vi "CSM-MassData Cache Status Viewer.vi"() -> ()   [LabVIEW 2017]
doc: "CSM Massdata cache status viewing tool that allows for an intuitive view of Massdata cache usage, helping to debug and optimize cache configuration.\n\n\n> [!NOTE] <b>CSM Massdata Argument Support</b>\n>\n> CSM Massdata argument support provides an efficient argument passing mechanism for transferring large amounts of data within CSM. By using a memory-efficient reference mechanism instead of direct data transfer, CSM Massdata improves the efficiency and performance of argument passing.\n> - The argument type defined by CSM Massdata is `<MassData>`, which can be obtained using the CSM - Argument Type VI.\n> - Data transmission of CSM Massdata is completely lossless. However, it is not suitable for storing data that requires indefinite persistence.\n>\n> <b>Note</b>: CSM Massdata internally uses a circular buffer mechanism. All CSM modules within the same application share the same Massdata buffer space. When the buffer is full, new data will overwrite old data starting from the beginning. Therefore, you need to set a reasonable buffer size to ensure that data is not overwritten before use, avoiding data loss."
uses:
  addons/MassData-Parameter/_support/FGV-MassData(lvlibp).vi
  addons/MassData-Parameter/CSM MassData Parameter Support.lvlib
panel:
  in  "CacheSize(Byte)":u32 format="%.0p"
  in  "Remove all Configurations":bool
  out "Write":cluster{dbl, dbl}(slide)={287840.0, 276144.0} scale=1.0..100000000.0 scale format="%#_6p"
  out "Read":cluster{dbl, dbl}(slide)={287840.0, 276144.0} scale=1.0..100000000.0 scale format="%#_6p"
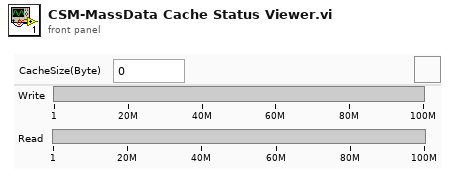
[diagram p1: front panel]
types:
  T1 = typedef "CSM MassData Parameter Support.lvlib/Def-MassDataOper-Status.ctl" = cluster{"Start":i32, "Size":i32, "Total":i32}
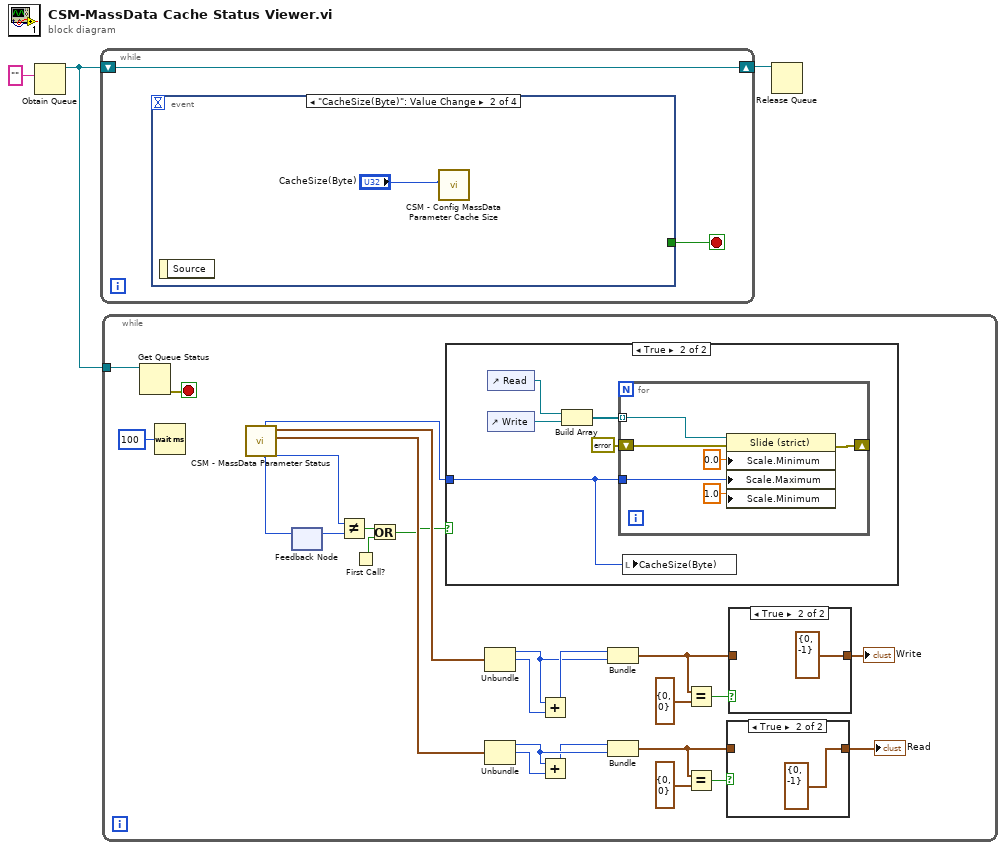
[diagram p0: block diagram]
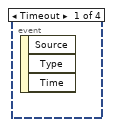
[diagram p2: hidden frame]
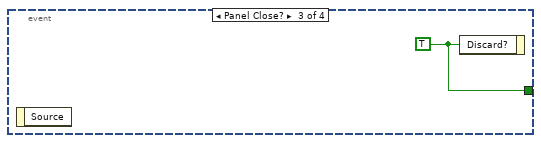
[diagram p3: hidden frame]
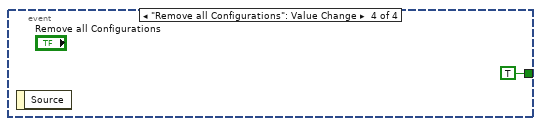
[diagram p4: hidden frame]
diagram:
  n1 = Obtain Queue(element data type="" ("name (unnamed)")) -> (queue out=w3:refnum<queue>)  [unwired: 4 in, 2 out]
  n2 = while {
    shift-right: [w4] -> w2
    shift-left: w3 -> [w4]
    stop <- w5 stop-if-true
    n3 = event shown="[1] \"CacheSize(Byte)\": Value Change" {
      selector: _ -> [_ _ _ _]
      dyn-events: _ -> [_ _ _ _]
      timeout: _ -> [_ _ _ _]
      tunnel: [_ _ w7 TRUE ("Discard?")] -> w5
      event Timeout {
        n4 = event-data() -> ()  [unwired: 1 in, 3 out]
      }
      event "CacheSize(Byte)": Value Change {
        n5 = event-data() -> ()  [unwired: 1 in, 1 out]
        n6 = call "CSM - Config MassData Parameter Cache Size.vi"("Size (1M)"="CacheSize(Byte)") -> ()  [unwired: 10 in, 1 out]
      }
      event Panel Close? {
        w7 = TRUE ("Discard?")
        n7 = event-data() -> ()  [unwired: 1 in, 1 out]
        n8 = event-data("Discard?"=w7) -> ()  [unwired: 1 in, 1 out]
      }
      event "Remove all Configurations": Value Change {
        n9 = event-data() -> ()  [unwired: 1 in, 1 out]
      }
    }
  }
  n10 = while {
    tunnel: w3 -> [w30]
    stop <- w31 stop-if-true
    n11 = Get Queue Status(queue=w30) -> (error out=w31:errorcluster)  [unwired: 2 in, 7 out]
    n12 = Wait (ms)(milliseconds to wait=u32 100) -> ()  [unwired: 1 out]
    n13 = call "CSM - MassData Parameter Status.vi"() -> ("Active Read Operation"=w28:T1, "Active Write Operation"=w29:T1, "Cache Size"=w19:i32)  [unwired: 7 in, 1 out]
    n14 = feedback #1() -> (w20:i32)  [unwired: 1 in]
    n15 = feedback-in #1(w19) -> ()
    n16 = Not Equal?(x=w19, y=w20) -> (x != y?=w21:bool)
    n17 = First Call?() -> (First Call?: T/F=w17:bool)
    n18 = Or(x=w21, y=w17) -> (x .or. y?=w18:bool)
    n19 = case shown="True" w18 {
      tunnel: w19 -> [_ w38]
      frame False {
      }
      frame True {
        n20 = control-ref of="Read"() -> (w41:refnum<vi>)
        n21 = control-ref of="Write"() -> (w40:refnum<vi>)
        n22 = Build Array(w41, w40) -> (w39:refnum<vi>[])
        n23 = for {
          tunnel: w38 -> [w47]
          shift-right: [w44] -> _
          shift-left: errorcluster {"status"=FALSE, "code"=0, "source"=""} ("error out") -> [w43]
          tunnel: w39 -> [w42] mode=indexing
          n24 = property on="Property Node" class="Slide (strict)"(reference=w42, error in=w43, "Scale.Minimum"=0.0 ("Scale.Range:Minimum"), "Scale.Maximum"=w47, "Scale.Minimum"=1.0 ("Scale.Range:Minimum")) -> (error out=w44:errorcluster)  [unwired: 1 out]
        }
        n25 = local write "CacheSize(Byte)"(w38) -> ()
      }
    }
    n26 = Unbundle(w29) -> ("Start"=w11:i32, "Size"=w13:i32)  [unwired: 1 out]
    n27 = Unbundle(w28) -> ("Start"=w16:i32, "Size"=w14:i32)  [unwired: 1 out]
    n28 = Add(x=w11, y=w13) -> (x+y=w12:i32)
    n29 = Add(x=w16, y=w14) -> (x+y=w15:i32)
    n30 = Bundle(w12, "Start"=w11) -> (w25:cluster{i32, "Start":i32})  [unwired: 1 in]
    n31 = Bundle(w15, "Start"=w16) -> (w24:cluster{i32, "Start":i32})  [unwired: 1 in]
    n32 = Equal?(x=w25, y=cluster{i32, "Start":i32} {0, "Start"=0}) -> (x = y?=w22:bool)
    n33 = Equal?(x=w24, y=cluster{i32, "Start":i32} {0, "Start"=0}) -> (x = y?=w23:bool)
    n34 = case shown="True" w23 {
      tunnel: w24 -> [w33 _]
      tunnel: [w33 cluster{i32, "Start":i32} {0, "Start"=-1}] -> w27
      frame False {
      }
      frame True {
      }
    }
    "Read" <- w27
    n35 = case shown="True" w22 {
      tunnel: [w35 cluster{i32, "Start":i32} {0, "Start"=-1}] -> w26
      tunnel: w25 -> [w35 _]
      frame False {
      }
      frame True {
      }
    }
    "Write" <- w26
  }
  n36 = Release Queue(queue=w2) -> ()  [unwired: 2 in, 3 out]
